vi "Bytes to DBL.vi"(11 "Bytes":u8[](array[numeric])) -> (3 "DBL":dbl)   [LabVIEW 2018, in "TCPServer.lvlib"]
uses:
  TCPServer.lvlib
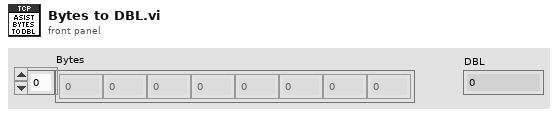
[diagram p1: front panel]
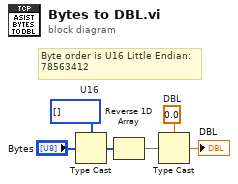
[diagram p0: block diagram]
diagram:
  w3 = 0.0  # DBL
  w6 = u16[] []  # U16
  # "Byte order is U16 Little Endian:\n78563412"
  n1 = Type Cast(type=w6, x="Bytes") -> (*(type *) &x=w5:u16[])
  n2 = Reverse 1D Array(array=w5) -> (reversed array=w4:u16[])
  n3 = Type Cast(type=w3, x=w4) -> (*(type *) &x=→"DBL":dbl)
